vi "VI-Create XControl.vi"(0 "Folder":path=path "C:/Users/hancock/Desktop", 7 "Name":string="Test", 11 "error in (no error)":errorcluster) -> (15 "error out":errorcluster)   [LabVIEW 2015]
uses:
  <vilib>/regexp/Match Regular Expression.xnode
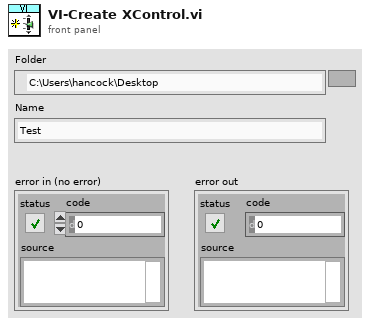
[diagram p1: front panel]
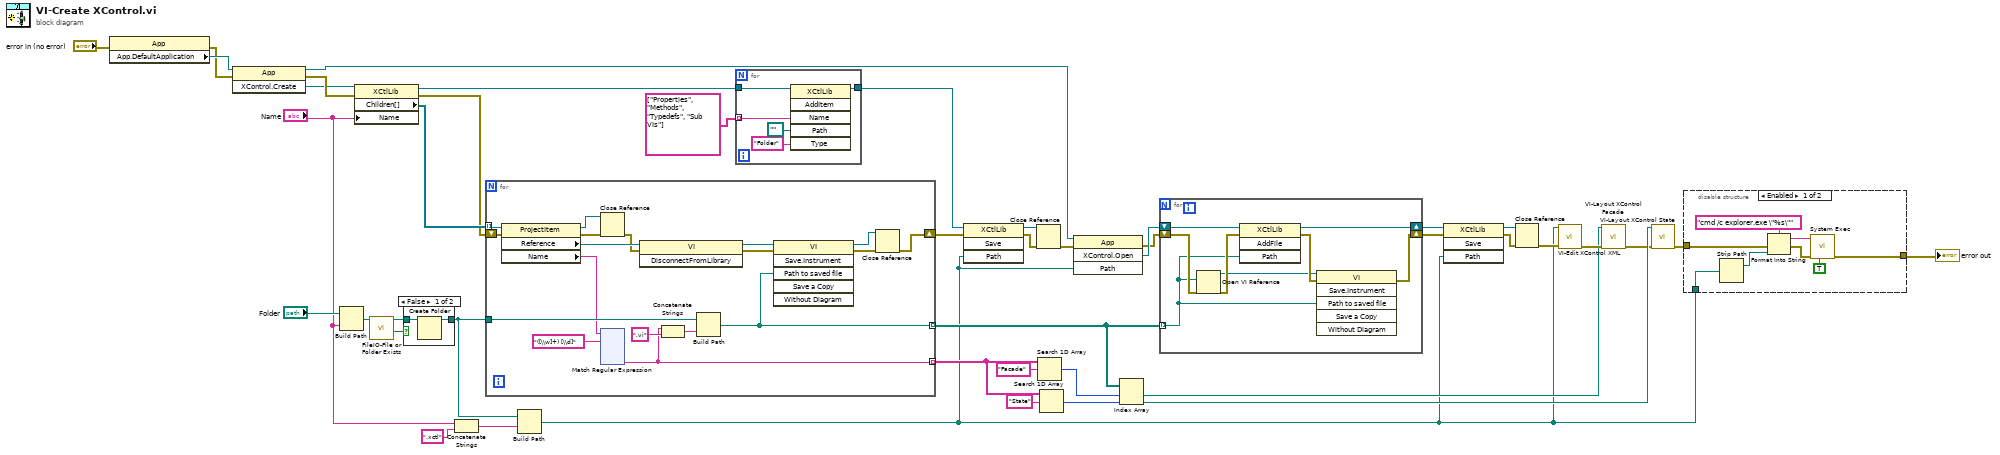
[diagram p0: block diagram]
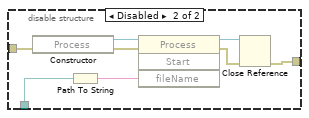
[diagram p2: hidden frame]
diagram:
  n1 = property class="App"(error in="error in (no error)") -> (error out=w3:errorcluster, "App.DefaultApplication"=w4:refnum<vi>)  [unwired: 1 in, 1 out]
  n2 = invoke class="App" method="XControl.Create"(reference=w4, error in=w3) -> (reference out=w5:refnum<vi>, error out=w27:errorcluster, "Create XControl"=w2:refnum<vi>)  [unwired: 1 in]
  n3 = Build Path(base path="Folder", name or relative path="Name") -> (appended path=w41:path)
  n4 = property class="XCtlLib"(reference=w2, error in=w27, "Name"="Name") -> (reference out=w37:refnum<vi>, error out=w31:errorcluster, "Children[]"=w43:refnum<vi>[])
  n5 = call "FileIO-File or Folder Exists.vi"("path"=w41) -> ("Exists?"=w39:bool, "dup path"=w40:path)  [unwired: 7 in, 2 out]
  n6 = case shown="False" w39 {
    tunnel: [w45 w46] -> w34
    tunnel: w40 -> [w44 w46]
    frame False {
      n7 = Create Folder(path (use dialog)=w44) -> (created path=w45:path)  [unwired: 2 in, 2 out]
    }
    frame True {
    }
  }
  n8 = Concatenate Strings("Name", ".xctl" ("string")) -> (w36:string)
  n9 = for {
    tunnel: w43 -> [w64] mode=indexing
    tunnel: w34 -> [w63]
    tunnel: [w48] -> w15 mode=indexing
    shift-right: [w49] -> w30
    shift-left: w31 -> [w55]
    tunnel: [w47] -> w12 mode=indexing
    n10 = property class="ProjectItem"(reference=w64, error in=w55) -> (reference out=w54:refnum<vi>, error out=w53:errorcluster, "Reference"=w61:refnum<vi>, "Name"=w57:string)
    n11 = Close Reference(reference=w54, error in (no error)=w53) -> (error out=w52:errorcluster)
    n12 = xnode "Match Regular Expression"("input string"=w57, "regular expression"="([\\w]+) [\\d]") -> ("submatch 1"=w47:string)  [unwired: 4 in, 5 out]
    n13 = invoke class="VI" method="DisconnectFromLibrary"(reference=w61, error in=w52) -> (reference out=w60:refnum<vi>, error out=w59:errorcluster)  [unwired: 1 in, 1 out]
    n14 = Concatenate Strings(w47, ".vi" ("string")) -> (w56:string)
    n15 = Build Path(base path=w63, name or relative path=w56) -> (appended path=w48:path)
    n16 = invoke class="VI" method="Save.Instrument"(reference=w60, error in=w59, "Path to saved file"=w48) -> (reference out=w51:refnum<vi>, error out=w50:errorcluster)  [unwired: 3 in, 4 out]
    n17 = Close Reference(reference=w51, error in (no error)=w50) -> (error out=w49:errorcluster)
  }
  n18 = Build Path(base path=w34, name or relative path=w36) -> (appended path=w1:path)
  n19 = for {
    tunnel: w37 -> [w185]
    tunnel: string[] ["Properties", "Methods", "Typedefs", "Sub VIs"] ("Name") -> [w182] mode=indexing
    tunnel: [w181] -> w32
    n20 = invoke class="XCtlLib" method="AddItem"(reference=w185, "Name"=w182, "Path"=path "", "Type"="Folder") -> (reference out=w181:refnum<vi>)  [unwired: 2 in, 5 out]
  }
  n21 = invoke class="XCtlLib" method="Save"(reference=w32, error in=w30, "Path"=w1) -> (reference out=w28:refnum<vi>, error out=w29:errorcluster)  [unwired: 1 in, 2 out]
  n22 = Close Reference(reference=w28, error in (no error)=w29) -> (error out=w26:errorcluster)
  n23 = Search 1D Array(1D array=w12, element="Facade") -> (index of element=w14:i32)  [unwired: 1 in]
  n24 = Search 1D Array(1D array=w12, element="State") -> (index of element=w10:i32)  [unwired: 1 in]
  n25 = invoke class="App" method="XControl.Open"(reference=w5, error in=w26, "Path"=w1) -> (error out=w22:errorcluster, "Open XControl"=w23:refnum<vi>)  [unwired: 1 in, 2 out]
  n26 = Index Array(array=w15, index #1=w14, index #2=w10) -> (element #1=w13:path, element #2=w8:path)
  n27 = for {
    shift-right: [w186] -> w24
    shift-left: w22 -> [w191]
    tunnel: w15 -> [w187] mode=indexing
    shift-right: [w192] -> w25
    shift-left: w23 -> [w193]
    n28 = Open VI Reference(vi path=w187, error in (no error)=w191) -> (vi reference=w188:refnum<vi>, error out=w190:errorcluster)  [unwired: 4 in]
    n29 = invoke class="XCtlLib" method="AddFile"(reference=w193, error in=w190, "Path"=w187) -> (reference out=w192:refnum<vi>, error out=w189:errorcluster)  [unwired: 1 in, 2 out]
    n30 = invoke class="VI" method="Save.Instrument"(reference=w188, error in=w189, "Path to saved file"=w187) -> (error out=w186:errorcluster)  [unwired: 3 in, 5 out]
  }
  n31 = invoke class="XCtlLib" method="Save"(reference=w25, error in=w24, "Path"=w1) -> (reference out=w21:refnum<vi>, error out=w20:errorcluster)  [unwired: 1 in, 2 out]
  n32 = Close Reference(reference=w21, error in (no error)=w20) -> (error out=w19:errorcluster)
  n33 = call "VI-Edit XControl XML.vi"("Path"=w1, "error in (no error)"=w19) -> ("error out"=w18:errorcluster)  [unwired: 13 in]
  n34 = call "VI-Layout XControl Facade.vi"("VI"=w13, "error in (no error)"=w18) -> ("error out"=w7:errorcluster)  [unwired: 13 in]
  n35 = call "VI-Layout XControl State.vi"("Path"=w8, "error in (no error)"=w7) -> ("error out"=w9:errorcluster)  [unwired: 13 in]
  n36 = disable-structure shown="Enabled" {
    disable-tunnel: w9 -> [w201 w202]
    disable-tunnel: [w200 w203] -> w6
    disable-tunnel: w1 -> [w194 w204]
    frame Enabled {
      n37 = Strip Path(path=w194) -> (stripped path=w195:path)  [unwired: 1 out]
      n38 = Format Into String(format string="cmd /c explorer.exe \"%s\"", error in=w201, w195) -> (resulting string=w198:string, error out=w196:errorcluster)  [unwired: 1 in]
      n39 = call <vilib>:"System Exec.vi"("run minimized? (F)"=TRUE, "error in (no error)"=w196, "command line"=w198) -> ("error out"=w200:errorcluster)  [unwired: 5 in, 3 out]
    }
    frame Disabled {
      n40 = constructor class="Process"(error in=w202) -> (reference out=w206:refnum<k24>, error out=w205:errorcluster)  [unwired: 2 in, 1 out]
      n41 = Path To String(path=w204) -> (string=w209:string)
      n42 = invoke class="Process" method="Start"(reference=w206, error in=w205, "fileName"=w209) -> (reference out=w208:refnum<k24>, error out=w207:errorcluster)  [unwired: 1 in, 2 out]
      n43 = Close Reference(reference=w208, error in (no error)=w207) -> (error out=w203:errorcluster)
    }
  }
  "error out" <- w6
